vi "Calculate Memory Addresses.vi"(0 ".hex lines":T1(array[cluster]), 11 "error in":errorcluster) -> (4 "Memory Address":u32[](array[numeric]), 8 "It's a Data Record Type":bool[](array[boolean]), 15 "error out":errorcluster)   [LabVIEW 2010]
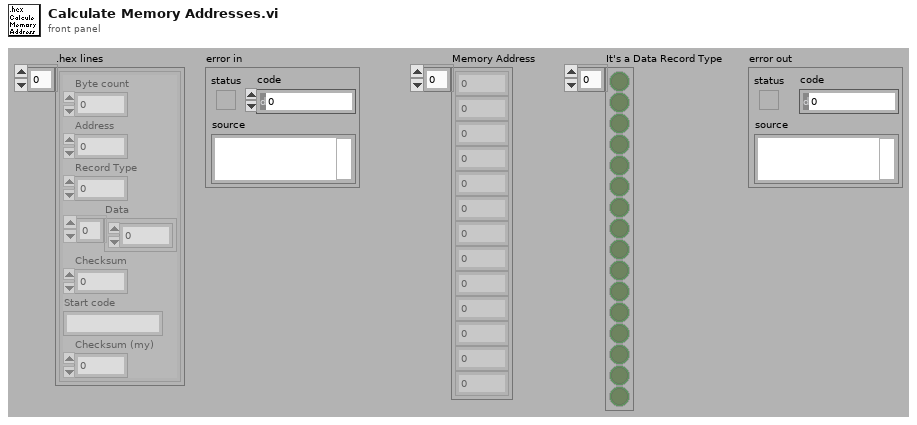
[diagram p1: front panel]
types:
  T1 = cluster{"Byte count":u8, "Address":u16, "Record Type":u8, "Data":u8[], "Checksum":u8, "Start code":string, "Checksum (my)":u8}[]
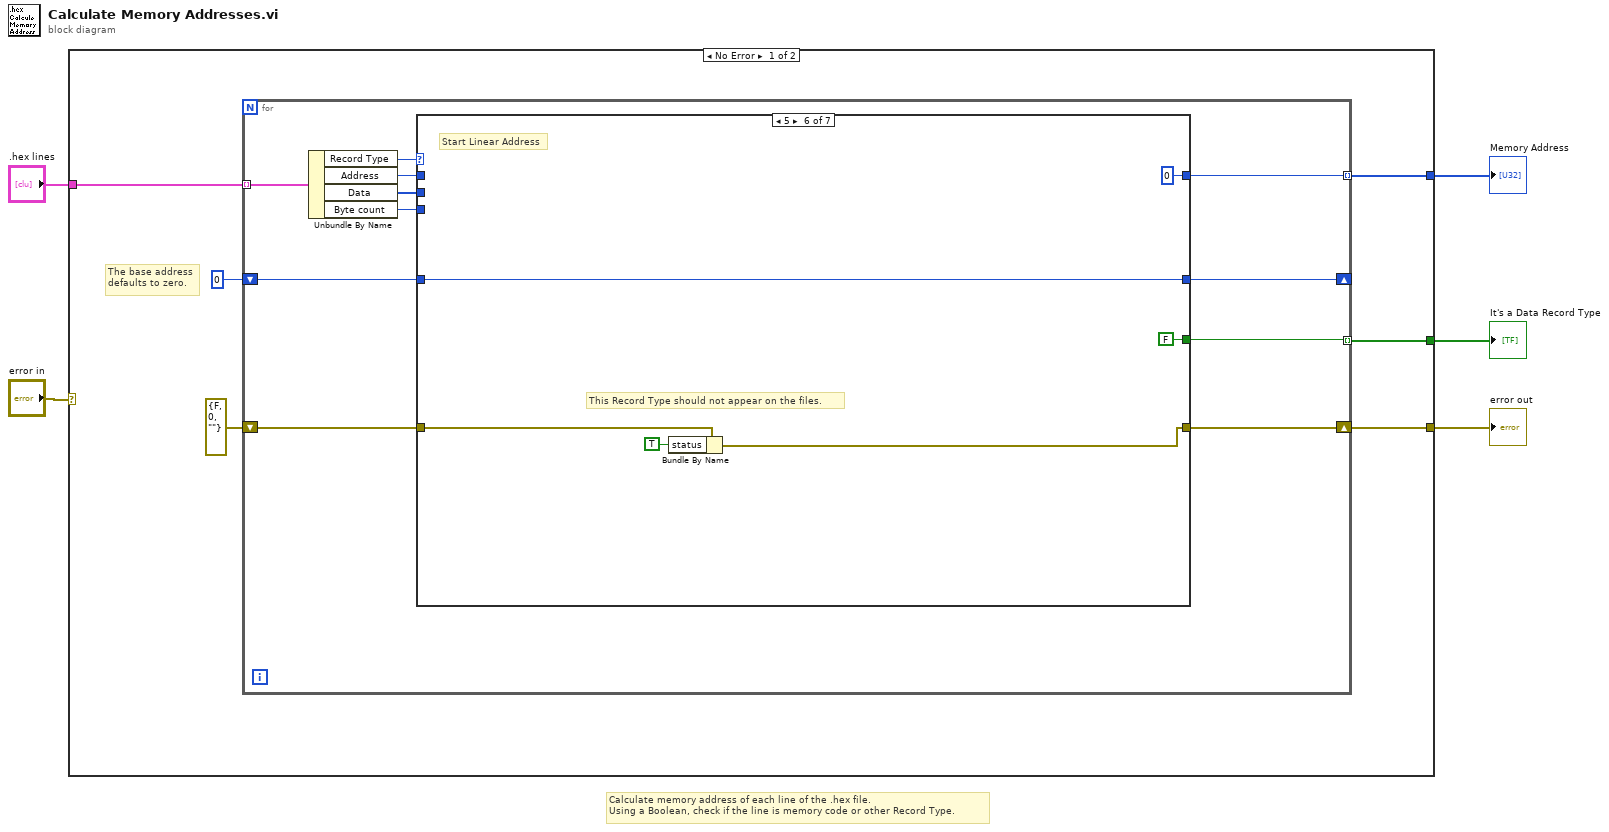
[diagram p0: block diagram]
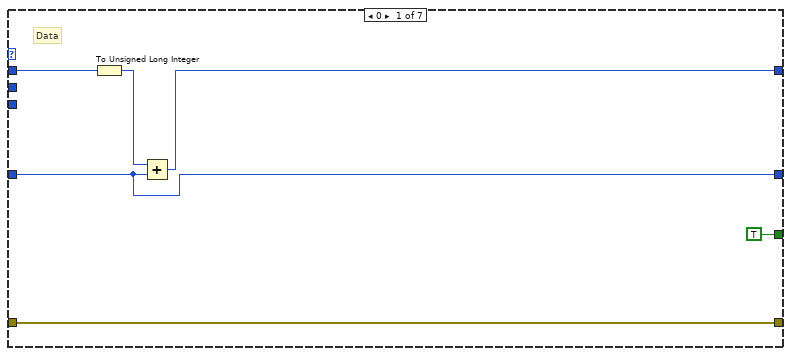
[diagram p2: hidden frame]
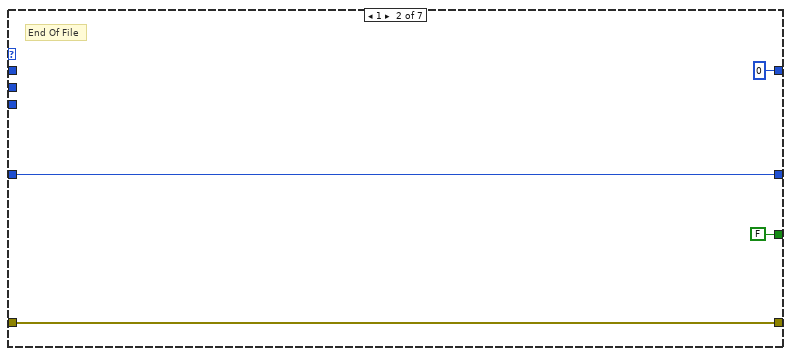
[diagram p3: hidden frame]
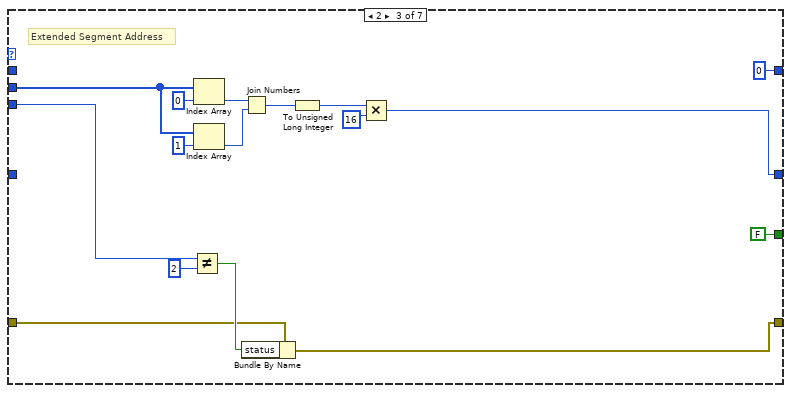
[diagram p4: hidden frame]
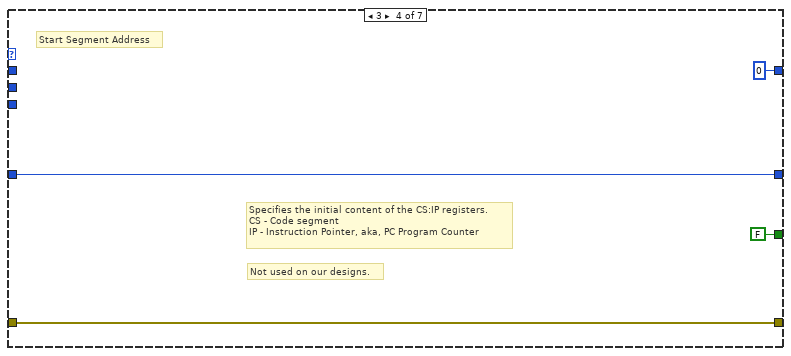
[diagram p5: hidden frame]
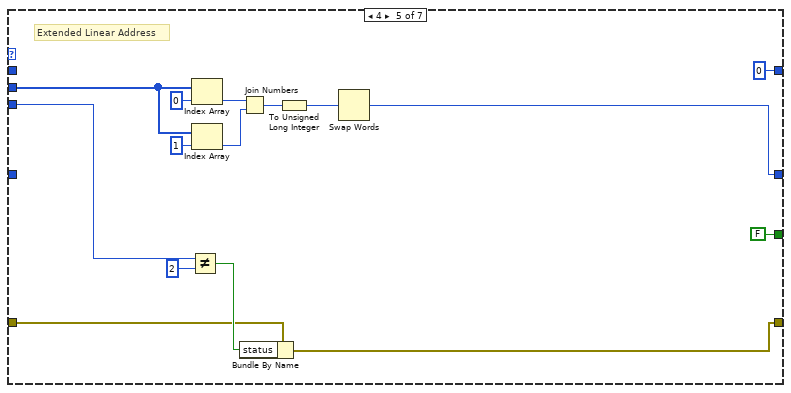
[diagram p6: hidden frame]
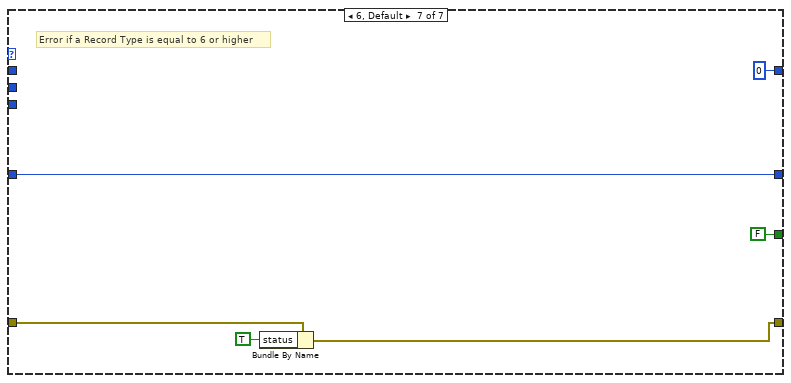
[diagram p7: hidden frame]
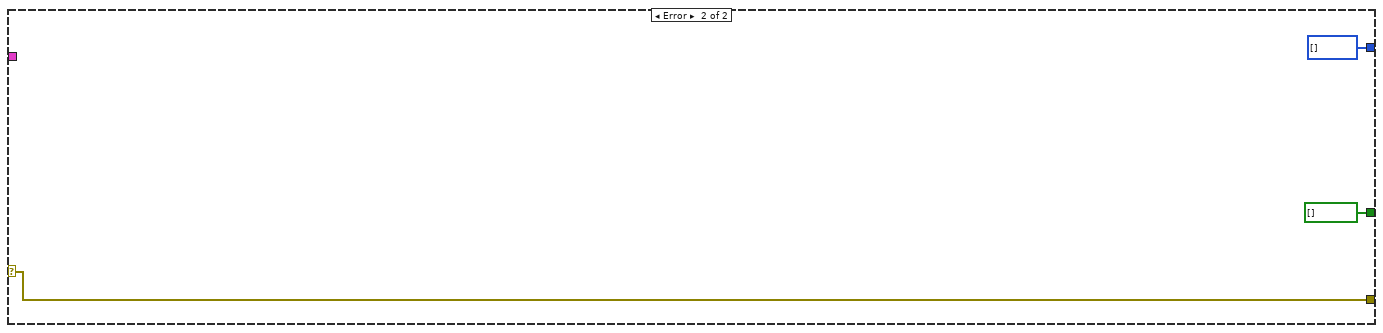
[diagram p8: hidden frame]
diagram:
  # "Calculate memory address of each line of the .hex file.\nUsing a Boolean, check if the line is memory code or other Record Type."
  n1 = case shown="No Error" "error in" {
    selector: "error in" -> [_ w82]
    tunnel: ".hex lines" -> [w9 _]
    tunnel: [w8 w82] -> w3
    tunnel: [w7 u32[] []] -> w4
    tunnel: [w6 bool[] []] -> w5
    frame No Error {
      # "The base address\ndefaults to zero."
      n2 = for {
        tunnel: w9 -> [w22] mode=indexing
        shift-right: [w14] -> _
        shift-left: u32 0 ("Data") -> [w20]
        tunnel: [w18] -> w7 mode=indexing
        shift-right: [w16] -> w8
        shift-left: errorcluster {"status"=FALSE, "code"=0, "source"=""} ("error out") -> [w17]
        tunnel: [w12] -> w6 mode=indexing
        n3 = Unbundle By Name(w22) -> ("Record Type"=w21:u8, "Address"=w19:u16, "Data"=w15:u8[], "Byte count"=w13:u8)
        n4 = case shown="5" w21 {
          tunnel: w20 -> [w24 w32 _ w52 _ w70 w76]
          tunnel: w19 -> [w28 _ _ _ _ _ _]
          tunnel: [w23 u32 0 ("Address") u32 0 ("Address") u32 0 ("Address") u32 0 ("Address") u32 0 ("Address") u32 0 ("Address")] -> w18
          tunnel: w17 -> [w27 w31 w38 w49 w56 w72 w78]
          tunnel: [w27 w31 w37 w49 w55 w71 w77] -> w16
          tunnel: w15 -> [_ _ w40 _ w65 _ _]
          tunnel: [w24 w32 w34 w52 w60 w70 w76] -> w14
          tunnel: w13 -> [_ _ w39 _ w59 _ _]
          tunnel: [TRUE ("status") FALSE ("status") FALSE ("status") FALSE ("status") FALSE ("status") FALSE ("status") FALSE ("status")] -> w12
          frame 0 {
            # "Data"
            n5 = To Unsigned Long Integer(number=w28) -> (unsigned 32bit integer=w25:u32)
            n6 = Add(x=w25, y=w24) -> (x+y=w23:u32)
          }
          frame 1 {
            # "End Of File"
          }
          frame 2 {
            # "Extended Segment Address"
            n7 = Not Equal?(x=w39, y=u8 2) -> (x != y?=w41:bool)
            n8 = Index Array(array=w40, index=0) -> (element=w43:u8)
            n9 = Index Array(array=w40, index=1) -> (element=w44:u8)
            n10 = Join Numbers(hi=w43, lo=w44) -> ((hi.lo)=w36:u16)
            n11 = Bundle By Name(cluster=w38, "status"=w41) -> (w37:errorcluster)
            n12 = To Unsigned Long Integer(number=w36) -> (unsigned 32bit integer=w33:u32)
            n13 = Multiply(x=w33, y=u32 16) -> (x*y=w34:u32)
          }
          frame 3 {
            # "Not used on our designs."
            # "Specifies the initial content of the CS:IP registers.\nCS - Code segment\nIP - Instruction Pointer, aka, PC Program Counter"
            # "Start Segment Address"
          }
          frame 4 {
            # "Extended Linear Address"
            n14 = Not Equal?(x=w59, y=u8 2) -> (x != y?=w57:bool)
            n15 = Index Array(array=w65, index=0) -> (element=w63:u8)
            n16 = Index Array(array=w65, index=1) -> (element=w64:u8)
            n17 = Join Numbers(hi=w63, lo=w64) -> ((hi.lo)=w62:u16)
            n18 = Bundle By Name(cluster=w56, "status"=w57) -> (w55:errorcluster)
            n19 = To Unsigned Long Integer(number=w62) -> (unsigned 32bit integer=w61:u32)
            n20 = Swap Words(1:w61) -> (0:w60:u32)
          }
          frame 5 {
            # "This Record Type should not appear on the files."
            # "Start Linear Address"
            n21 = Bundle By Name(cluster=w72, "status"=TRUE) -> (w71:errorcluster)
          }
          frame 6, Default {
            # "Error if a Record Type is equal to 6 or higher"
            n22 = Bundle By Name(cluster=w78, "status"=TRUE) -> (w77:errorcluster)
          }
        }
      }
    }
    frame Error {
    }
  }
  "error out" <- w3
  "Memory Address" <- w4
  "It's a Data Record Type" <- w5
